vi "Average - Original.vi"() -> ()   [LabVIEW 2012]
panel:
  out "x/y 4":dbl
  out "x/y 3":dbl
  out "x/y 2":dbl
  out "x/y":dbl
  out "size(s)":i32
  out "Izlaz iz Bool Niza":u32=16
  in  "Sekvenca":dbl[](array[numeric])
  in  "Treshold":dbl=0.8
  in  "stop":bool
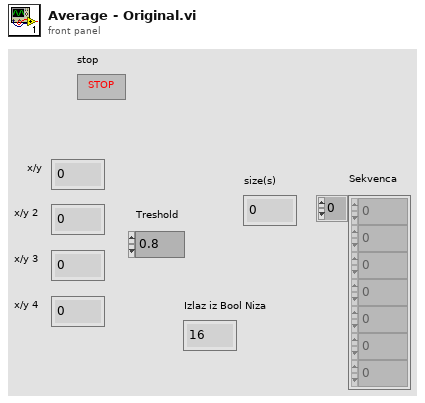
[diagram p1: front panel]
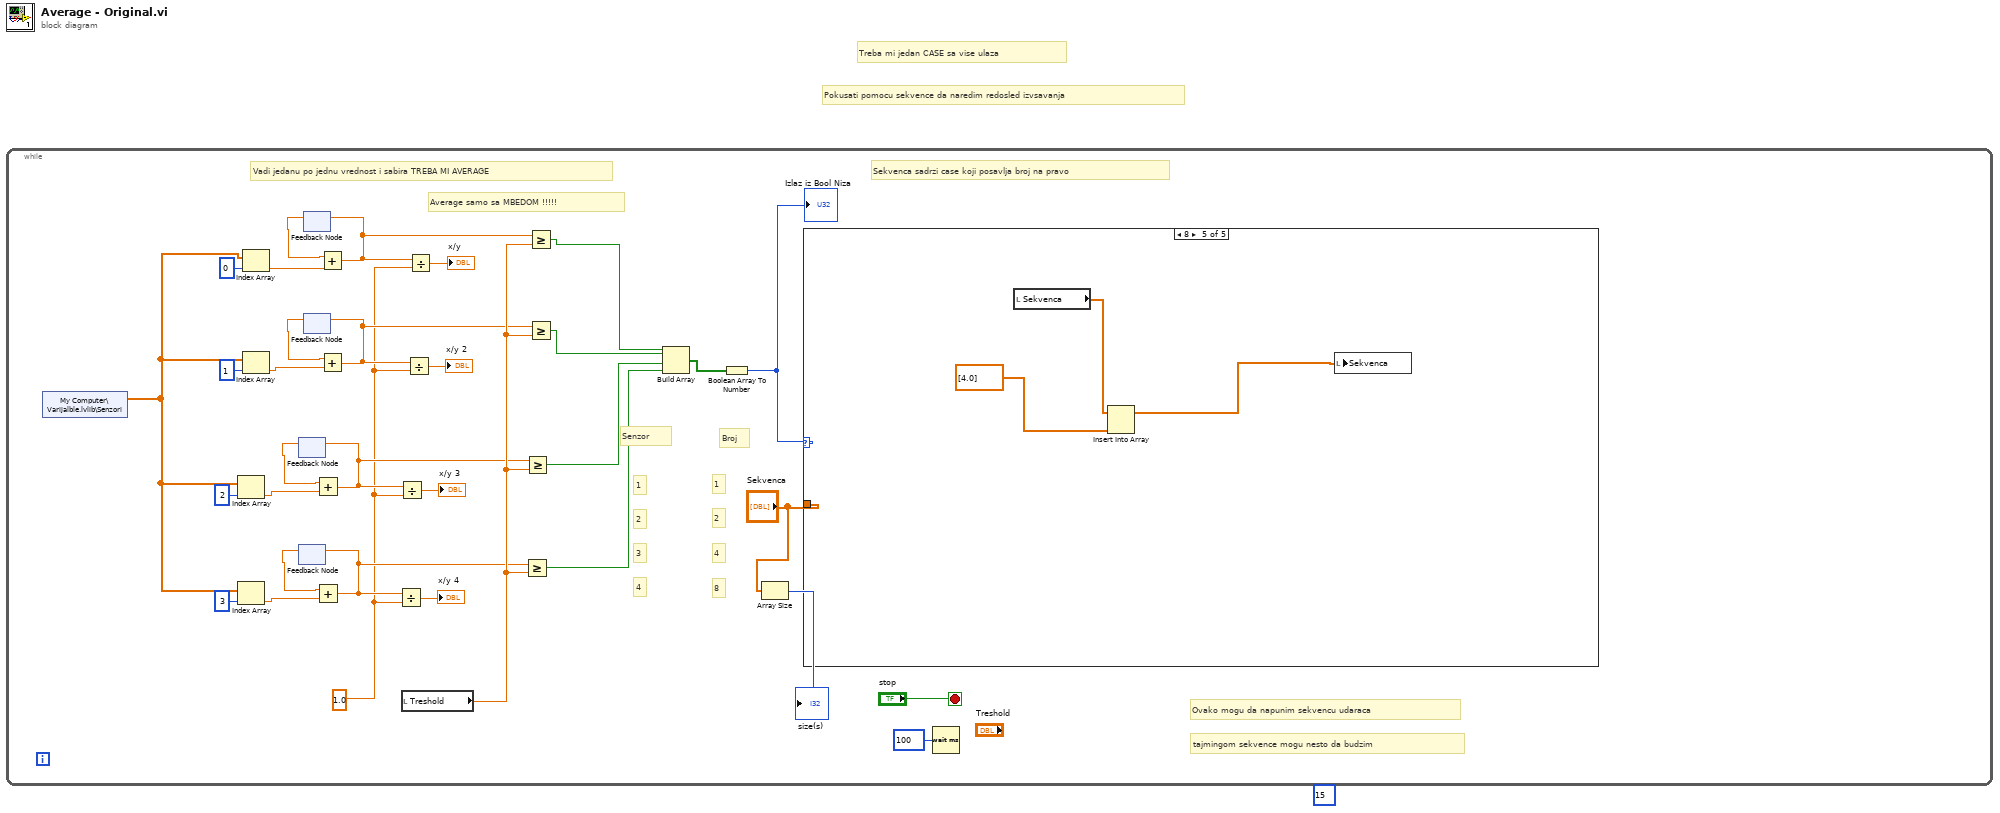
[diagram p0: block diagram]
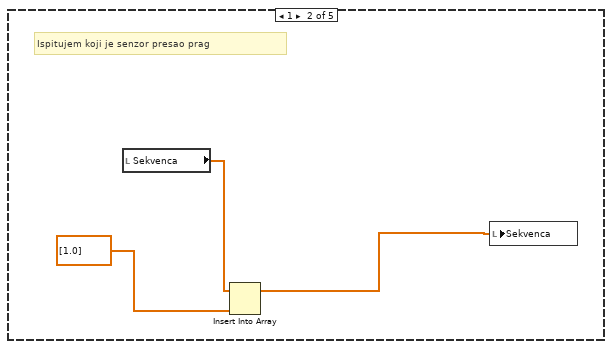
[diagram p3: hidden frame]
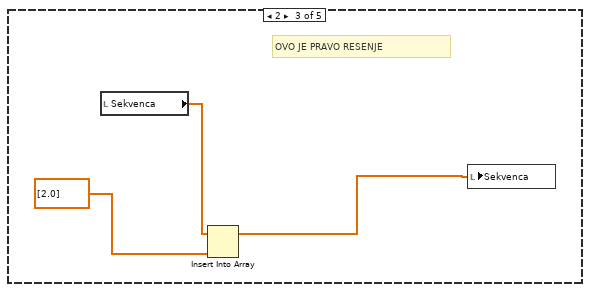
[diagram p4: hidden frame]
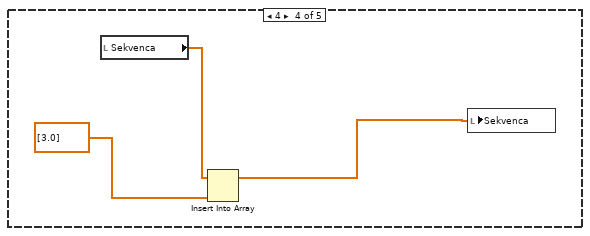
[diagram p5: hidden frame]
diagram:
  (unwired) u32 15 ("number")
  # "Pokusati pomocu sekvence da naredim redosled izvsavanja"
  # "Treba mi jedan CASE sa vise ulaza"
  n1 = while {
    stop <- "stop" stop-if-true
    w6 = 1.0 ("y")
    # "8"
    # "4"
    # "2"
    # "1"
    # "4"
    # "3"
    # "2"
    # "1"
    # "Broj"
    # "Senzor"
    # "Sekvenca sadrzi case koji posavlja broj na pravo"
    # "tajmingom sekvence mogu nesto da budzim"
    # "Ovako mogu da napunim sekvencu udaraca"
    # "Average samo sa MBEDOM !!!!!"
    # "Vadi jedanu po jednu vrednost i sabira TREBA MI AVERAGE"
    n2 = shared-variable "My Computer\\Varijalble.lvlib\\Senzori"() -> (w1:dbl[])  [unwired: 1 in, 1 out]
    n3 = Index Array(array=w1, index=2) -> (element=w3:dbl)
    n4 = Index Array(array=w1, index=3) -> (element=w2:dbl)
    n5 = Index Array(array=w1, index=0) -> (element=w5:dbl)
    n6 = Index Array(array=w1, index=1) -> (element=w4:dbl)
    n7 = feedback #1() -> (w26:dbl)  [unwired: 1 in]
    n8 = feedback #2() -> (w24:dbl)  [unwired: 1 in]
    n9 = feedback #3() -> (w30:dbl)  [unwired: 1 in]
    n10 = feedback #4() -> (w28:dbl)  [unwired: 1 in]
    n11 = Add(x=w26, y=w3) -> (x+y=w12:dbl)
    n12 = feedback-in #1(w12) -> ()
    n13 = Add(x=w24, y=w2) -> (x+y=w11:dbl)
    n14 = feedback-in #2(w11) -> ()
    n15 = Add(x=w30, y=w5) -> (x+y=w14:dbl)
    n16 = feedback-in #3(w14) -> ()
    n17 = Add(x=w28, y=w4) -> (x+y=w13:dbl)
    n18 = feedback-in #4(w13) -> ()
    n19 = Divide(x=w11, y=w6) -> (x/y=→"x/y 4":dbl)
    n20 = Divide(x=w12, y=w6) -> (x/y=→"x/y 3":dbl)
    n21 = local read "Treshold"() -> (w23:dbl)
    n22 = Divide(x=w13, y=w6) -> (x/y=→"x/y 2":dbl)
    n23 = Divide(x=w14, y=w6) -> (x/y=→"x/y":dbl)
    n24 = Greater Or Equal?(x=w11, y=w23) -> (x >= y?=w19:bool)
    n25 = Greater Or Equal?(x=w12, y=w23) -> (x >= y?=w20:bool)
    n26 = Greater Or Equal?(x=w14, y=w23) -> (x >= y?=w22:bool)
    n27 = Greater Or Equal?(x=w13, y=w23) -> (x >= y?=w21:bool)
    n28 = Build Array(w22, w21, w20, w19) -> (w18:bool[])
    n29 = Boolean Array To Number(Boolean array=w18) -> (number=w17:u32)
    "Izlaz iz Bool Niza" <- w17
    n30 = Array Size(array="Sekvenca") -> (size(s)=→"size(s)":i32)
    n31 = case shown="8" w17 {
      tunnel: "Sekvenca" -> [_ _ _ _ _]
      frame 0, Default {
      }
      frame 1 {
        # "Ispitujem koji je senzor presao prag"
        n32 = local read "Sekvenca"() -> (w34:dbl[])
        n33 = Insert Into Array(array=w34, new element=dbl[] [1.0]) -> (w36:dbl[])  [unwired: 1 in]
        n34 = local write "Sekvenca"(w36) -> ()
      }
      frame 2 {
        # "OVO JE PRAVO RESENJE"
        n35 = local read "Sekvenca"() -> (w37:dbl[])
        n36 = Insert Into Array(array=w37, new element=dbl[] [2.0]) -> (w39:dbl[])  [unwired: 1 in]
        n37 = local write "Sekvenca"(w39) -> ()
      }
      frame 4 {
        n38 = local read "Sekvenca"() -> (w40:dbl[])
        n39 = Insert Into Array(array=w40, new element=dbl[] [3.0]) -> (w42:dbl[])  [unwired: 1 in]
        n40 = local write "Sekvenca"(w42) -> ()
      }
      frame 8 {
        n41 = local read "Sekvenca"() -> (w43:dbl[])
        n42 = Insert Into Array(array=w43, new element=dbl[] [4.0]) -> (w45:dbl[])  [unwired: 1 in]
        n43 = local write "Sekvenca"(w45) -> ()
      }
    }
    n44 = Wait (ms)(milliseconds to wait=u32 100) -> ()  [unwired: 1 out]
  }
